vi "as DBL.vi"(11 "bytes":u8[](array[numeric]) format="%b") -> (3 "DBL":dbl)   [LabVIEW 2020, in "MessagePack.lvlib" / "MessagePackNumeric.lvclass"]
uses:
  MessagePackNumeric.lvclass
  MessagePackNumeric.lvclass/MessagePackNumeric.ctl
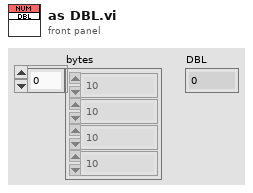
[diagram p1: front panel]
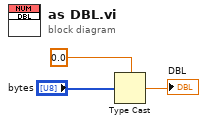
[diagram p0: block diagram]
diagram:
  n1 = Type Cast(type=0.0 ("INT8"), x="bytes") -> (*(type *) &x=→"DBL":dbl)
